vi "AndorCameraSwitch.vi"(8 "error in (no error)":errorcluster, 10 "Andor Camera":bool, 11 "HWConfiguration in":refnum<class "HWConfiguration.lvclass">) -> (0 "error out":errorcluster, 3 "HWConfiguration out":refnum<class "HWConfiguration.lvclass">)   [LabVIEW 2009, in "Hardware.lvlib" / "HWControllers.lvlib" / "HWConfiguration.lvclass"]
uses:
  HWConfiguration.lvclass
  HWConfiguration.lvclass/HWConfiguration.ctl
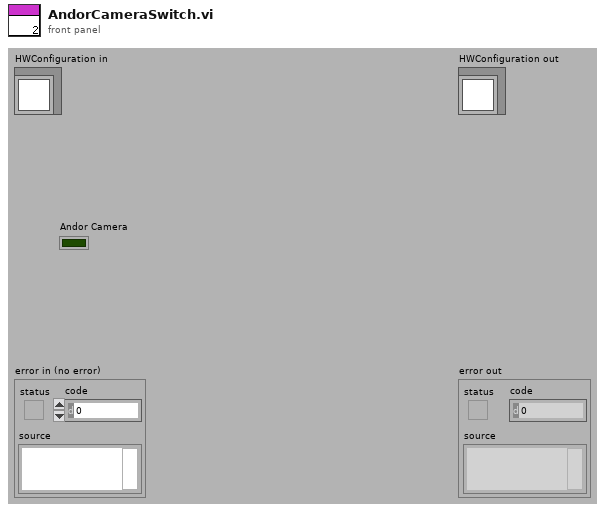
[diagram p1: front panel]
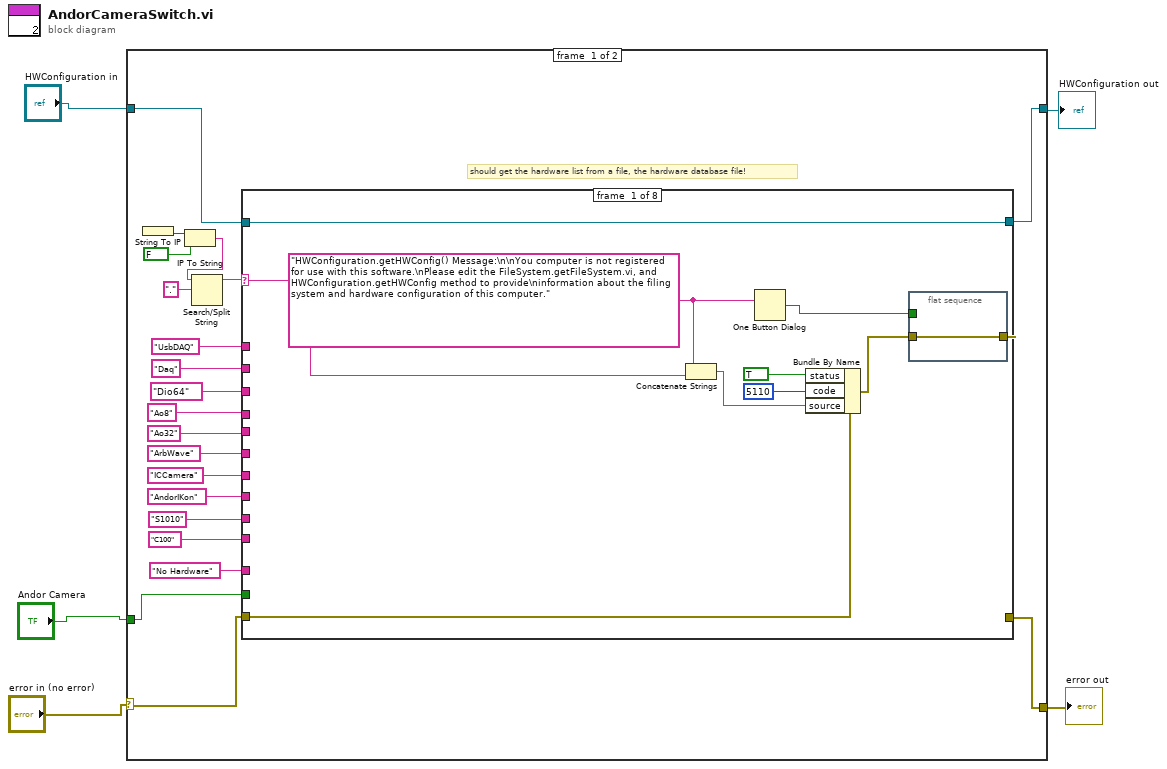
[diagram p0: block diagram]
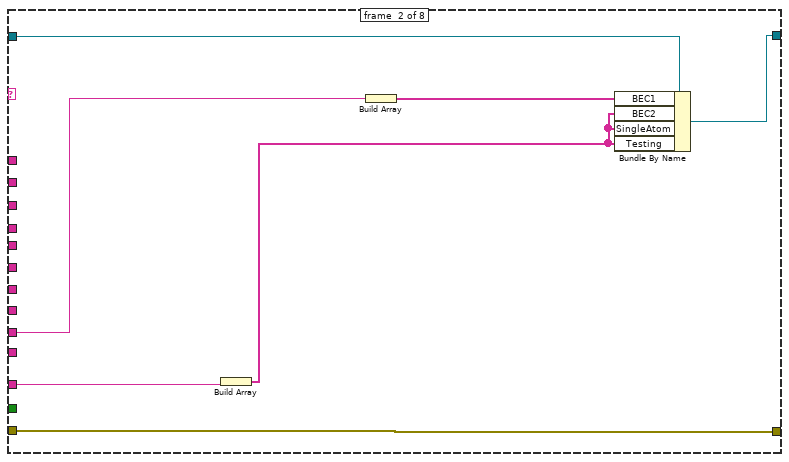
[diagram p2: hidden frame]
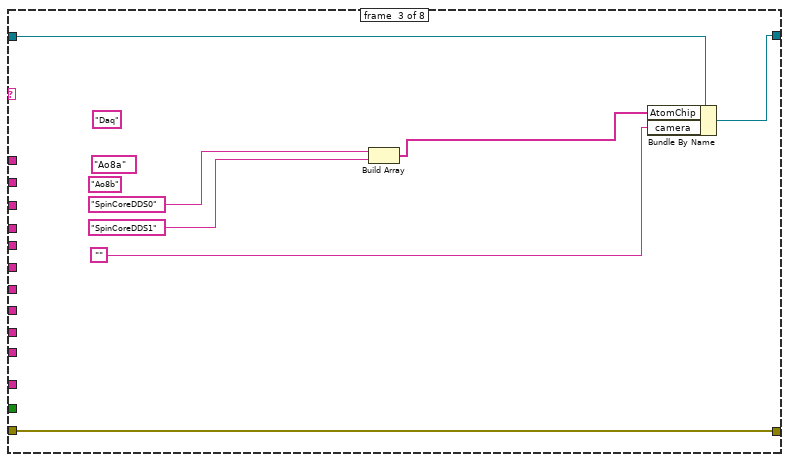
[diagram p3: hidden frame]
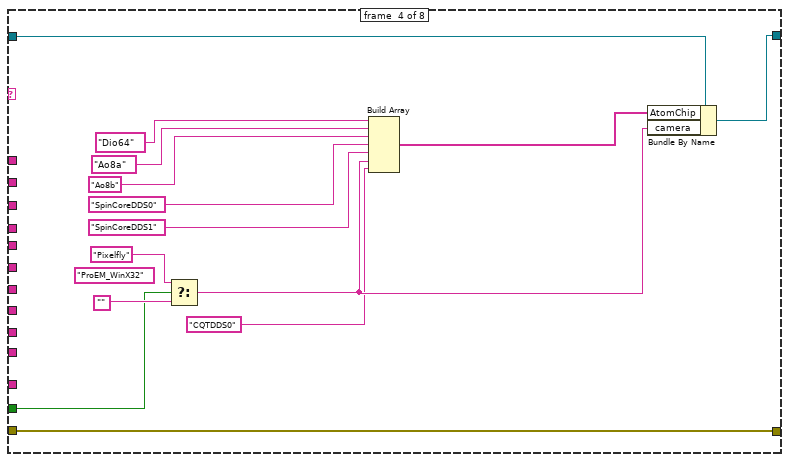
[diagram p4: hidden frame]
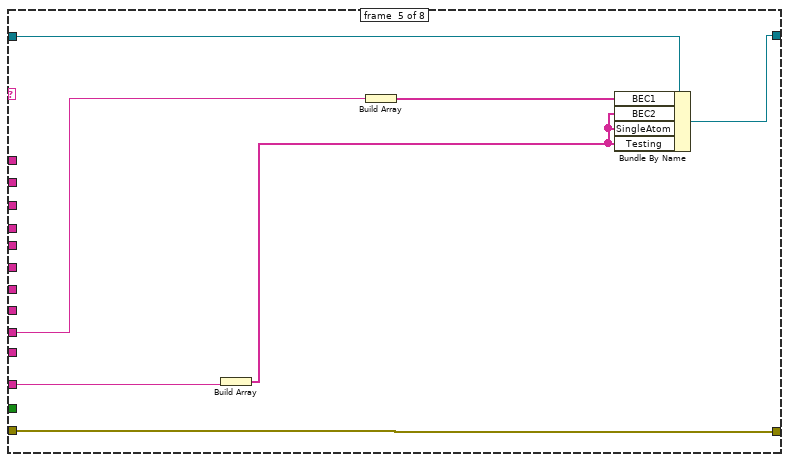
[diagram p5: hidden frame]
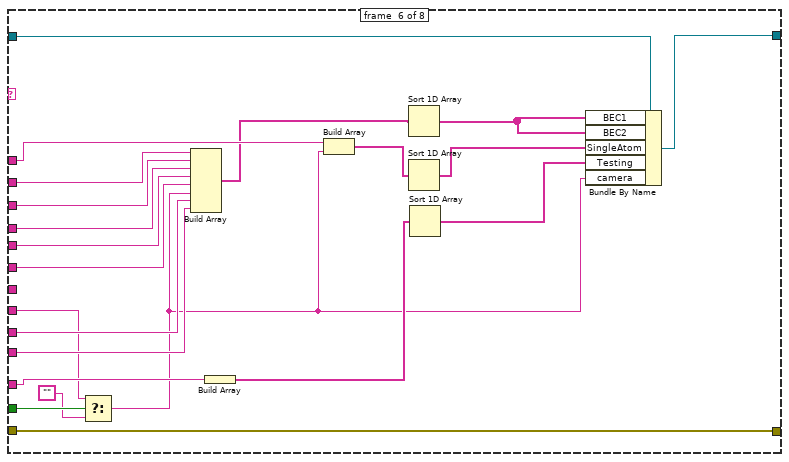
[diagram p6: hidden frame]
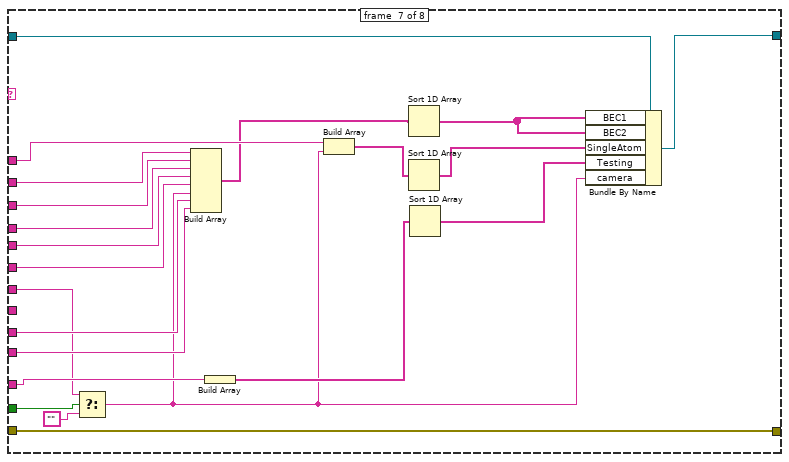
[diagram p7: hidden frame]
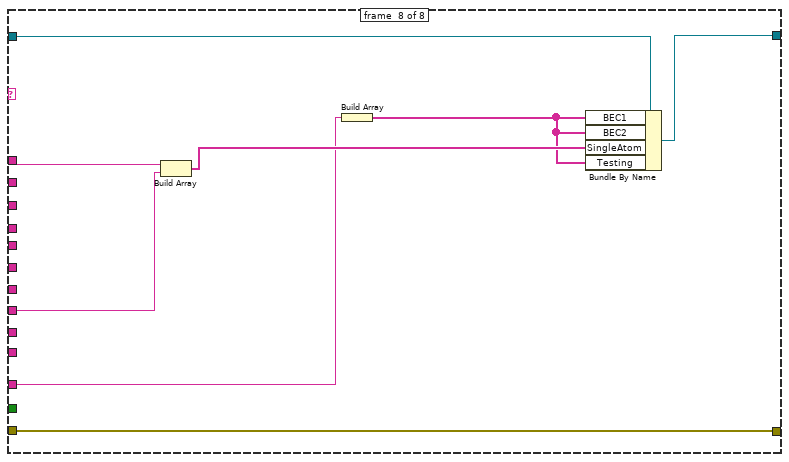
[diagram p8: hidden frame]
diagram:
  n1 = case shown="No Error" "error in (no error)" {
    selector: "error in (no error)" -> [w21 w126]
    tunnel: [w18 w126] -> w3
    tunnel: [w19 w125] -> w2
    tunnel: "HWConfiguration in" -> [w20 w125]
    tunnel: "Andor Camera" -> [w6 _]
    frame #0 {
      # "should get the hardware list from a file, the hardware database file!"
      n2 = String To IP() -> (0:w25:u32)  [unwired: 1 in]
      n3 = IP To String(1:FALSE, 2:w25) -> (0:w23:string)
      n4 = Search/Split String(string=w23, search string/char (-)=".") -> (substring before match=w22:string)  [unwired: 1 in, 2 out]
      n5 = case shown="\"DCTX52S\"" w22 {
        selector: w22 -> [w30 _ _ _ _ _ _ _]
        tunnel: w20 -> [w27 w43 w49 w65 w71 w93 w115 w123]
        tunnel: [w27 w42 w46 w63 w70 w92 w114 w122] -> w19
        tunnel: w21 -> [w28 w44 w45 w62 w72 w94 w116 w124]
        tunnel: [w33 w44 w45 w62 w72 w94 w116 w124] -> w18
        tunnel: "UsbDAQ" -> [_ _ _ _ _ w84 w106 w121]
        tunnel: "Daq" -> [_ _ _ _ _ w91 w113 _]
        tunnel: "Dio64" -> [_ _ _ _ _ w77 w99 _]
        tunnel: "Ao8" -> [_ _ _ _ _ w90 w112 _]
        tunnel: "Ao32" -> [_ _ _ _ _ w89 w111 _]
        tunnel: "ArbWave" -> [_ _ _ _ _ w88 w110 _]
        tunnel: "ICCamera" -> [_ _ _ _ _ _ w96 _]
        tunnel: "AndorIKon" -> [_ _ _ _ _ w75 _ w120]
        tunnel: "S1010" -> [_ w39 _ _ w67 w87 w109 _]
        tunnel: "C100" -> [_ _ _ _ _ w86 w108 _]
        tunnel: "No Hardware" -> [_ w41 _ _ w69 w85 w107 w117]
        tunnel: w6 -> [_ _ _ w57 _ w76 w98 _]
        frame #0 {
          w31 = "HWConfiguration.getHWConfig() Message:\n\nYou computer is not registered for use with this software.\nPlease edit the FileSystem.getFileSystem.vi, and HWConfiguration.getHWConfig method to provide\ninformation about the filing system and hardware configuration of this computer."
          n6 = Concatenate Strings(w31, w30) -> (w29:string)
          n7 = One Button Dialog(message=w31) -> (true=w32:bool)  [unwired: 1 in]
          n8 = Bundle By Name(cluster=w28, "status"=TRUE, "code"=5110, "source"=w29) -> (w34:errorcluster)
          n9 = flat-sequence {
            tunnel: w34 -> [w37]
            tunnel: [w37] -> w33
            tunnel: w32 -> [_]
            frame #0 {
            }
          }
        }
        frame #1 {
          n10 = Build Array(w41) -> (w40:string[])
          n11 = Build Array(w39) -> (w38:string[])
          n12 = Bundle By Name(cluster=w43, "BEC1"=w38, "BEC2"=w40, "SingleAtom"=w40, "Testing"=w40) -> (w42:refnum<class "HWConfiguration.lvclass">)
        }
        frame #2 {
          (unwired) "Ao8b"
          (unwired) "Ao8a"
          (unwired) "Daq"
          n13 = Build Array("SpinCoreDDS0", "SpinCoreDDS1") -> (w47:string[])
          n14 = Bundle By Name(cluster=w49, "AtomChip"=w47, "camera"="") -> (w46:refnum<class "HWConfiguration.lvclass">)
        }
        frame #3 {
          (unwired) "ProEM_WinX32"
          n15 = Select(t="Pixelfly", s=w57, f="") -> (s? t:f=w55:string)
          n16 = Build Array("Dio64", "Ao8a", "Ao8b", "SpinCoreDDS0", "SpinCoreDDS1", w55, "CQTDDS0") -> (w64:string[])
          n17 = Bundle By Name(cluster=w65, "AtomChip"=w64, "camera"=w55) -> (w63:refnum<class "HWConfiguration.lvclass">)
        }
        frame #4 {
          n18 = Build Array(w69) -> (w68:string[])
          n19 = Build Array(w67) -> (w66:string[])
          n20 = Bundle By Name(cluster=w71, "BEC1"=w66, "BEC2"=w68, "SingleAtom"=w68, "Testing"=w68) -> (w70:refnum<class "HWConfiguration.lvclass">)
        }
        frame #5 {
          n21 = Select(t=w75, s=w76, f="") -> (s? t:f=w73:string)
          n22 = Build Array(w91, w77, w90, w89, w88, w73, w87, w86) -> (w83:string[])
          n23 = Build Array(w85) -> (w79:string[])
          n24 = Build Array(w84, w73) -> (w81:string[])
          n25 = Sort 1D Array(array=w83) -> (sorted array=w82:string[])
          n26 = Sort 1D Array(array=w81) -> (sorted array=w80:string[])
          n27 = Sort 1D Array(array=w79) -> (sorted array=w78:string[])
          n28 = Bundle By Name(cluster=w93, "BEC1"=w82, "BEC2"=w82, "SingleAtom"=w80, "Testing"=w78, "camera"=w73) -> (w92:refnum<class "HWConfiguration.lvclass">)
        }
        frame #6 {
          n29 = Select(t=w96, s=w98, f="") -> (s? t:f=w95:string)
          n30 = Build Array(w113, w99, w112, w111, w110, w95, w109, w108) -> (w105:string[])
          n31 = Build Array(w107) -> (w101:string[])
          n32 = Build Array(w106, w95) -> (w103:string[])
          n33 = Sort 1D Array(array=w105) -> (sorted array=w104:string[])
          n34 = Sort 1D Array(array=w103) -> (sorted array=w102:string[])
          n35 = Sort 1D Array(array=w101) -> (sorted array=w100:string[])
          n36 = Bundle By Name(cluster=w115, "BEC1"=w104, "BEC2"=w104, "SingleAtom"=w102, "Testing"=w100, "camera"=w95) -> (w114:refnum<class "HWConfiguration.lvclass">)
        }
        frame #7 {
          n37 = Build Array(w121, w120) -> (w119:string[])
          n38 = Build Array(w117) -> (w118:string[])
          n39 = Bundle By Name(cluster=w123, "BEC1"=w118, "BEC2"=w118, "SingleAtom"=w119, "Testing"=w118) -> (w122:refnum<class "HWConfiguration.lvclass">)
        }
      }
    }
    frame #1 {
    }
  }
  "error out" <- w3
  "HWConfiguration out" <- w2
